vi "Main.vi"() -> ()   [LabVIEW 2014]
uses:
  <vilib>/userdefined/High Color/IMAQdx.ctl
  <vilib>/myRIO/Common/Instrument Driver Framework/myRIO v1.0/UART/vis/myRIO v1.0 Close UART.vi
  <vilib>/addons/control/pid/pid.llb/PID (DBL).vi
  <vilib>/myRIO/Common/Instrument Driver Framework/Utilities/vis/FPGA Ref Manager.vi
  <vilib>/myRIO/Common/Instrument Driver Framework/myRIO v1.0/myRIO v1.0 Reset FPGA.vi
  <vilib>/myRIO/Common/Instrument Driver Framework/myRIO v1.0/IRQ/vis/myRIO v1.0 IRQ Info FGV.vi
  <vilib>/myRIO/Common/Instrument Driver Framework/myRIO v1.0/IRQ/vis/myRIO v1.0 Timer IRQ Info FGV.vi
  <vilib>/myRIO/Common/Instrument Driver Framework/myRIO v1.0/IRQ/vis/myRIO v1.0 ISR Agent.vi
  <vilib>/vision/driver/NI_Vision_Acquisition_Software.lvlib
  <vilib>/vision/NI_Vision_Development_Module.lvlib
  <vilib>/myRIO/Instrument Drivers/Utilities/Utilities.lvlib
  <vilib>/addons/control/pid/NI_PID_pid.lvlib
panel:
  out "pwm elbow":dbl
  in  "PID gains 2":T1={"proportional gain (Kc)"=1.0, "integral time (Ti, min)"=0.01, "derivative time (Td, min)"=0.0} {"derivative time (Td, min)" format="%.3f"; "integral time (Ti, min)" format="%.3f"; "proportional gain (Kc)" format="%.3f"}
  out "pid elbow":dbl
  out "Boolean 4":bool
  out "Boolean 3":bool
  out "Numeric 2":dbl
  out "Numeric":dbl
  out "pid base":dbl
  out "pwm base":dbl
  out "Boolean 2":bool
  out "Boolean":bool
  in  "PID gains":T1={"proportional gain (Kc)"=0.001, "integral time (Ti, min)"=-0.001, "derivative time (Td, min)"=0.001} {"derivative time (Td, min)" format="%.3f"; "integral time (Ti, min)" format="%.3f"; "proportional gain (Kc)" format="%.3f"}
  out "error out":errorcluster
  in  "Red or Hue Range":cluster{dbl, dbl}(slide)={0.0, 73.71681415929203} scale=0.0..255.0
  in  "Green or Sat Range":cluster{dbl, dbl}(slide)={159.1907514450867, 255.0} scale=0.0..255.0
  out "live feed":T2(plugin-control)
  out "Number of Objects":i32
  out "Found Objects":T3(array[cluster]) {"Aspect Ratio" format="%.2f"; "Orientation" format="%.2f"; "Area" format="%.2f"; "Object Center"."Y" format="%.2f"; "Object Center"."X" format="%.2f"}
  out "Largest Area":sgl
  out "Object Info":T4
  in  "Blue or Luma or Val or Inten Range":cluster{dbl, dbl}(slide)={34.638728323699425, 255.0} scale=0.0..255.0
  in  "stop":bool
  out "threshold":T2(plugin-control)
  in  "Number of Erosion":i32=2
  out "centroid x-displacement":sgl
  out "centroid y-displacement":sgl
  out "Left x-displacement":i32
  out "Top y-displacement":i32
  out "Right x-displacement":i32
  out "Bottom y-displacement":i32
  out "object width":i32
  out "object height":i32
  out "duty cycle of wrist motor":dbl format="%.2f"
  out "box area":dbl
  in  "Session In":T5
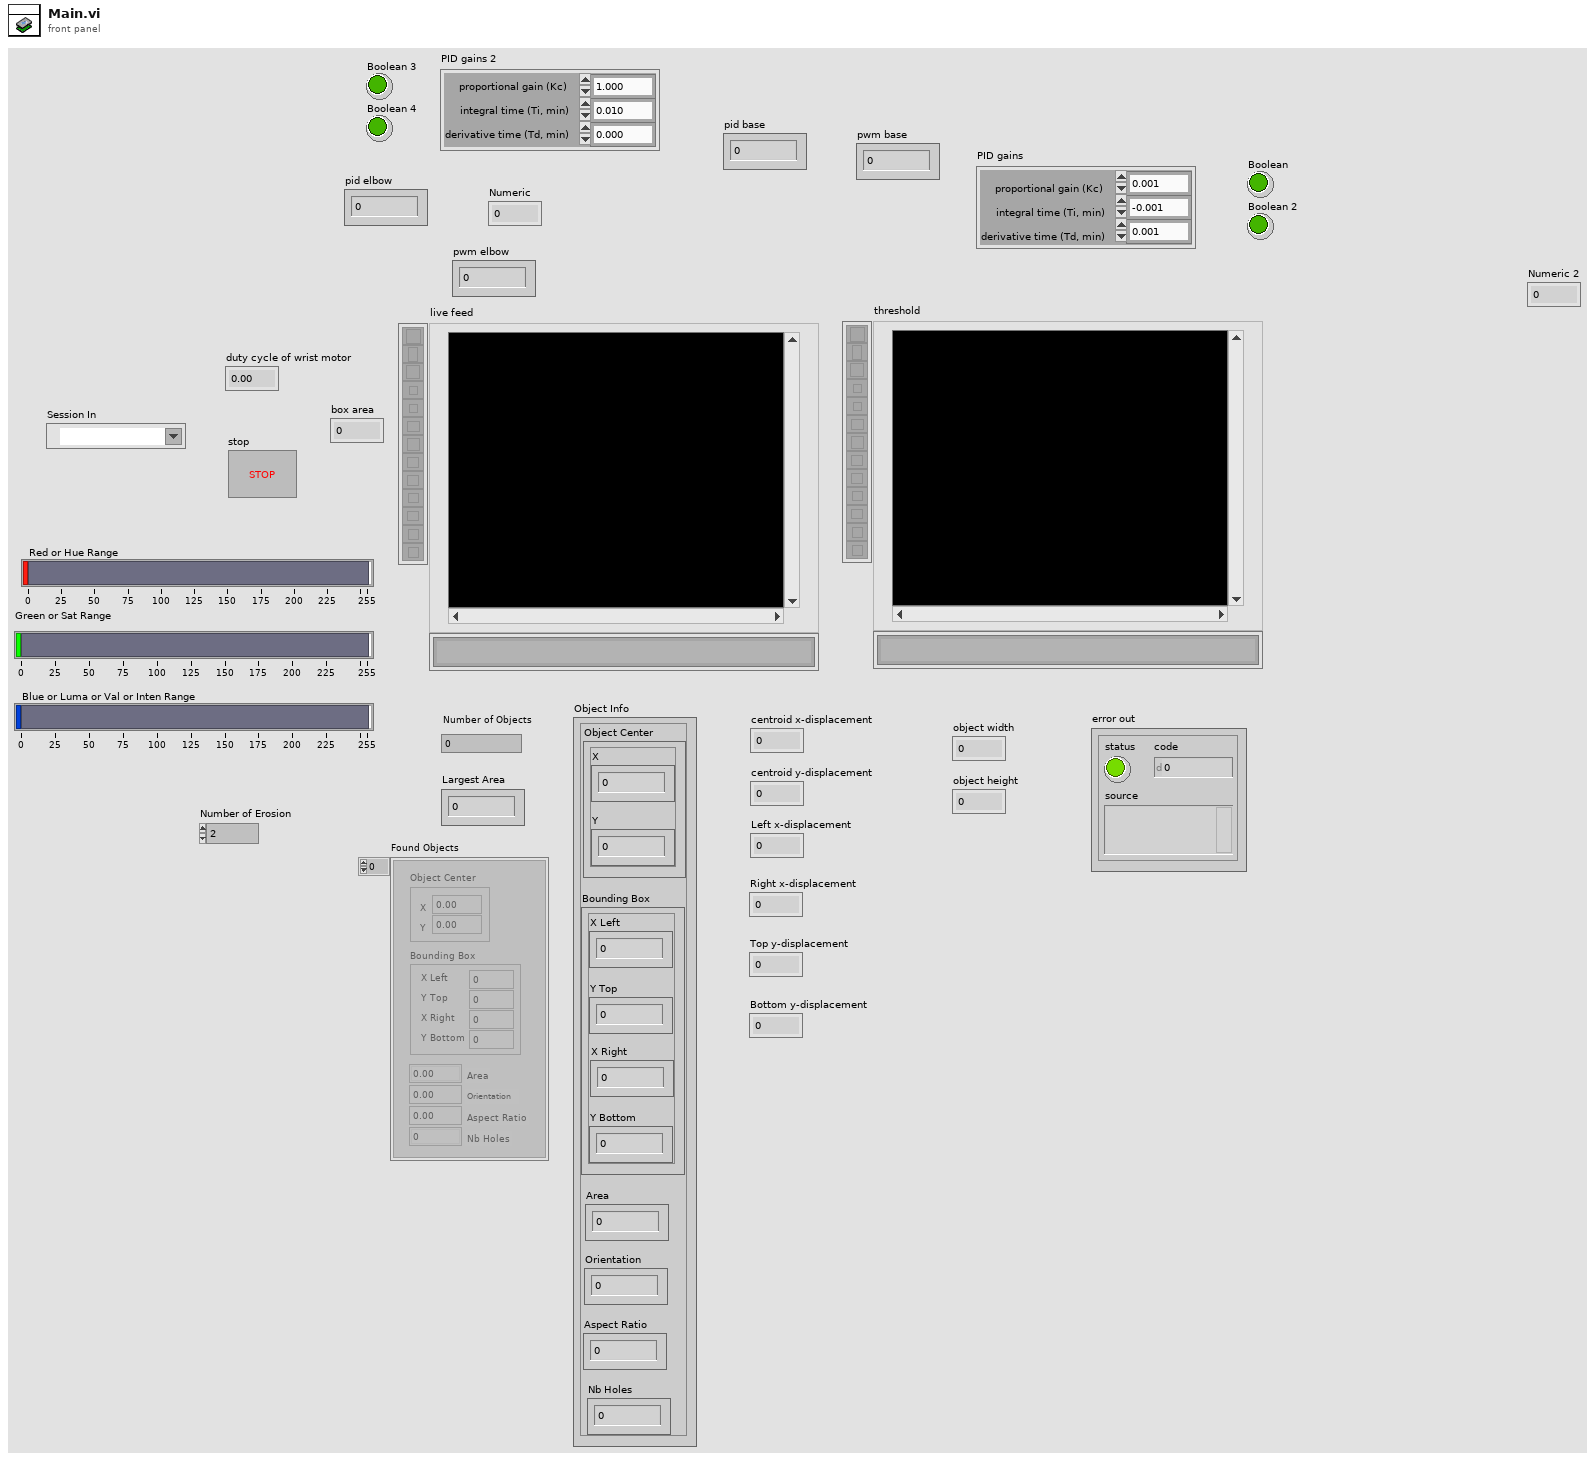
[diagram p1: front panel]
types:
  T1 = cluster{"proportional gain (Kc)":dbl, "integral time (Ti, min)":dbl, "derivative time (Td, min)":dbl}
  T2 = typedef "IMAQ Image.ctl" = refnum<image>
  T3 = cluster{"Object Center":cluster{"X":sgl, "Y":sgl}, "Bounding Box":cluster{"X Left":i32, "Y Top":i32, "X Right":i32, "Y Bottom":i32}, "Area":sgl, "Orientation":sgl, "Aspect Ratio":sgl, "Nb Holes":i32}[]
  T4 = cluster{"Object Center":cluster{"X":sgl, "Y":sgl}, "Bounding Box":cluster{"X Left":i32, "Y Top":i32, "X Right":i32, "Y Bottom":i32}, "Area":sgl, "Orientation":sgl, "Aspect Ratio":sgl, "Nb Holes":i32}
  T5 = typedef "IMAQdx.ctl" = refnum<k21>
  T6 = cluster{"Objects":u16, "Threshold":i32, "Reject Border":bool, "Fill Holes":bool, "Min Object Size":bool, "Min Size":i32, "Max Object Size":bool, "Max Size":i32, "Show Search Area":bool, "Show Center":bool, "Show Bounding Box":bool}
  T7 = typedef "Image Type" = u32
  T8 = cluster{"X Left":i32, "Y Top":i32, "X Right":i32, "Y Bottom":i32}
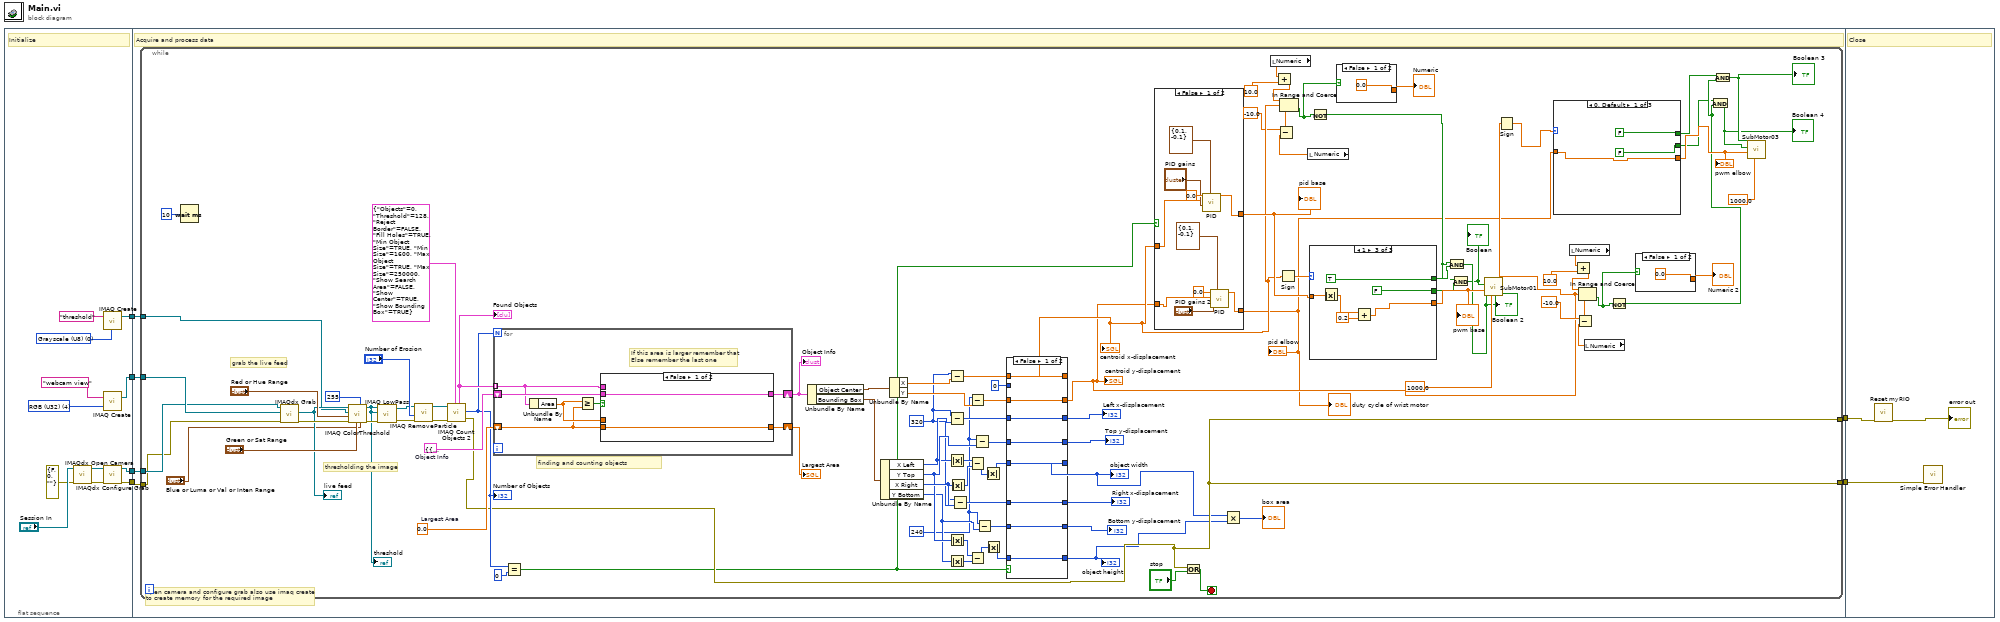
[diagram p0: block diagram]
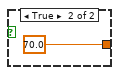
[diagram p2: hidden frame]
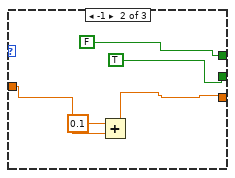
[diagram p3: hidden frame]
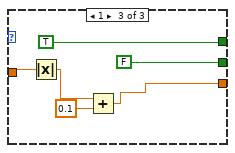
[diagram p4: hidden frame]
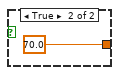
[diagram p5: hidden frame]
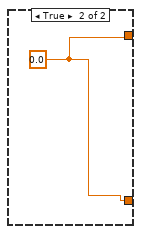
[diagram p6: hidden frame]
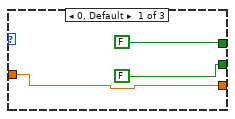
[diagram p7: hidden frame]
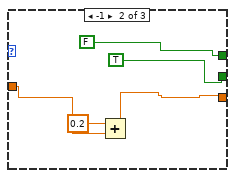
[diagram p8: hidden frame]
diagram:
  n1 = flat-sequence {
    tunnel: [w16] -> w6
    tunnel: [w13] -> w5
    tunnel: [w10] -> w4
    tunnel: [w7] -> w3
    tunnel: [w20] -> w2
    tunnel: w6 -> [w23]
    tunnel: [w19] -> w1
    tunnel: w5 -> [w22]
    tunnel: w4 -> [w21]
    tunnel: w3 -> [w24]
    tunnel: w2 -> [w188]
    tunnel: w1 -> [w186]
    frame #0 {
      w8 = T7 0 items=["Grayscale (U8)", "Grayscale (I16)", "Grayscale (SGL)", "Complex (CSG)", "RGB (U32)", "HSL (U32)", "RGB (U64)", "Grayscale (U16)"] ("Image Type")
      w17 = T7 4 items=["Grayscale (U8)", "Grayscale (I16)", "Grayscale (SGL)", "Complex (CSG)", "RGB (U32)", "HSL (U32)", "RGB (U64)", "Grayscale (U16)"] ("Image Type")
      # "Initialize"
      n2 = call <vilib>:"IMAQdx Open Camera.vi"("error in"=errorcluster {"status"=FALSE, "code"=0, "source"=""} ("error out"), "Session In"="Session In") -> ("error out"=w12:errorcluster, "Session Out"=w14:T5)  [unwired: 8 in]
      n3 = call "IMAQ Create"("Image Name"="threshold", "Image Type"=w8) -> ("New Image"=w7:T2)  [unwired: 3 in, 1 out]
      n4 = call "IMAQ Create"("Image Name"="webcam view", "Image Type"=w17) -> ("New Image"=w16:T2)  [unwired: 3 in, 1 out]
      n5 = call <vilib>:"IMAQdx Configure Grab.vi"("error in"=w12, "Session In"=w14) -> ("error out"=w10:errorcluster, "Session Out"=w13:T5)  [unwired: 8 in]
    }
    frame #1 {
      # "open camera and configure grab also use imaq create \nto create memory for the required image"
      # "Acquire and process data"
      n6 = while {
        tunnel: w24 -> [w71]
        tunnel: w23 -> [w70]
        tunnel: w22 -> [w69]
        tunnel: w21 -> [w68]
        tunnel: [w65] -> w20
        tunnel: [w65] -> w19
        stop <- w66 stop-if-true
        w76 = 240
        w78 = 320
        w116 = T4 {"Object Center"={"X"=0.0, "Y"=0.0}, "Bounding Box"={"X Left"=0, "Y Top"=0, "X Right"=0, "Y Bottom"=0}, "Area"=0.0, "Orientation"=0.0, "Aspect Ratio"=0.0, "Nb Holes"=0}  # Object Info
        w115 = sgl 0.0  # Largest Area
        # "finding and counting objects"
        # "thresholding the image"
        # "grab the live feed"
        n7 = Wait (ms)(milliseconds to wait=u32 10) -> ()  [unwired: 1 out]
        n8 = call <vilib>:"IMAQdx Grab.vi"("error in"=w68, "Image In"=w70, "Session In"=w69) -> ("error out"=w122:errorcluster, "Image Out"=w118:T2)  [unwired: 5 in, 2 out]
        "live feed" <- w118
        n9 = call "IMAQ ColorThreshold"("Blue or Luma or Val or Inten Range"="Blue or Luma or Val or Inten Range", "Replace Value"=255, "Green or Sat Range"="Green or Sat Range", "error in (no error)"=w122, "Red or Hue Range"="Red or Hue Range", "Image Dst"=w71, "Image Src"=w118) -> ("error out"=w112:errorcluster, "Image Dst Out"=w111:T2)  [unwired: 3 in]
        "threshold" <- w111
        n10 = call "IMAQ LowPass"("Image Src"=w111, "Image Mask"=w111, "error in (no error)"=w112) -> ("Image Dst Out"=w73:T2, "error out"=w75:errorcluster)  [unwired: 4 in]
        n11 = call "IMAQ RemoveParticle"("error in (no error)"=w75, "Number of Erosion"="Number of Erosion", "Image Src"=w73) -> ("error out"=w74:errorcluster, "Image Dst Out"=w72:T2)  [unwired: 7 in]
        n12 = call "IMAQ Count Objects 2"("Settings"=T6 {"Objects"=0, "Threshold"=128, "Reject Border"=FALSE, "Fill Holes"=TRUE, "Min Object Size"=TRUE, "Min Size"=1600, "Max Object Size"=TRUE, "Max Size"=250000, "Show Search Area"=FALSE, "Show Center"=TRUE, "Show Bounding Box"=TRUE}, "error in (no error)"=w74, "Image"=w72) -> ("error out"=w65:errorcluster, "Number of Objects"=w104:i32, "Objects"=w117:T3)  [unwired: 4 in, 2 out]
        "Number of Objects" <- w104
        "Found Objects" <- w117
        n13 = for {
          N: w104 -> [_]
          tunnel: w117 -> [w178] mode=indexing
          shift-right: [w181] -> w114
          shift-left: w115 -> [w175]
          shift-right: [w180] -> w110
          shift-left: w116 -> [w179]
          # "If this area is larger remember that\nElse remember the last one"
          n14 = Unbundle By Name(w178) -> ("Area"=w177:sgl)
          n15 = Greater Or Equal?(x=w177, y=w175) -> (x >= y?=w176:bool)
          n16 = case shown="False" w176 {
            tunnel: [w183 w185] -> w181
            tunnel: w177 -> [_ w185]
            tunnel: w175 -> [w183 _]
            tunnel: [w182 w184] -> w180
            tunnel: w179 -> [w182 _]
            tunnel: w178 -> [_ w184]
            frame False {
            }
            frame True {
            }
          }
        }
        "Largest Area" <- w114
        "Object Info" <- w110
        n17 = Equal?(x=w104, y=0) -> (x = y?=w58:bool)
        n18 = Unbundle By Name(w110) -> ("Object Center"=w109:cluster{"X":sgl, "Y":sgl}, "Bounding Box"=w107:T8)
        n19 = Unbundle By Name(w107) -> ("X Left"=w79:i32, "Y Top"=w80:i32, "X Right"=w81:i32, "Y Bottom"=w77:i32)
        n20 = Unbundle By Name(w109) -> ("X"=w83:sgl, "Y"=w82:sgl)
        n21 = Subtract(x=w78, y=w83) -> (x-y=w97:sgl)
        n22 = Subtract(x=w78, y=w79) -> (x-y=w95:i32)
        n23 = Absolute Value(x=w79) -> (abs(x)=w89:i32)
        n24 = Absolute Value(x=w80) -> (abs(x)=w91:i32)
        n25 = Absolute Value(x=w77) -> (abs(x)=w90:i32)
        n26 = Absolute Value(x=w81) -> (abs(x)=w88:i32)
        n27 = Subtract(x=w78, y=w81) -> (x-y=w93:i32)
        n28 = Subtract(x=w76, y=w82) -> (x-y=w96:sgl)
        n29 = Subtract(x=w89, y=w88) -> (x-y=w87:i32)
        n30 = Subtract(x=w91, y=w90) -> (x-y=w85:i32)
        n31 = Subtract(x=w76, y=w80) -> (x-y=w94:i32)
        n32 = Subtract(x=w76, y=w77) -> (x-y=w92:i32)
        n33 = Absolute Value(x=w87) -> (abs(x)=w86:i32)
        n34 = Absolute Value(x=w85) -> (abs(x)=w84:i32)
        n35 = case shown="False" w58 {
          tunnel: [w173 w174] -> w56
          tunnel: 0 -> [_ w174]
          tunnel: [w172 w174] -> w33
          tunnel: [w171 w174] -> w101
          tunnel: [w169 w174] -> w100
          tunnel: [w170 w174] -> w99
          tunnel: [w168 w174] -> w98
          tunnel: w97 -> [w173 _]
          tunnel: w96 -> [w172 _]
          tunnel: w95 -> [w171 _]
          tunnel: w94 -> [w170 _]
          tunnel: w93 -> [w169 _]
          tunnel: w92 -> [w168 _]
          tunnel: [w167 w174] -> w63
          tunnel: w86 -> [w167 _]
          tunnel: [w166 w174] -> w62
          tunnel: w84 -> [w166 _]
          frame False {
          }
          frame True {
          }
        }
        "centroid x-displacement" <- w56
        "centroid y-displacement" <- w33
        "Left x-displacement" <- w101
        "Top y-displacement" <- w99
        "Right x-displacement" <- w100
        "Bottom y-displacement" <- w98
        "object width" <- w63
        "object height" <- w62
        n36 = case shown="False" w58 {
          tunnel: [w142 w151] -> w32
          tunnel: w33 -> [w145 _]
          tunnel: [w143 w151] -> w57
          tunnel: w56 -> [w144 _]
          frame False {
            n37 = call-poly <vilib>:"PID.vi"("output range"=cluster{"output high":dbl, "output low":dbl} {"output high"=0.1, "output low"=-0.1}, "PID gains"="PID gains", "process variable"=w144, "setpoint"=0.0) -> ("output"=w143:dbl)  [unwired: 6 in, 1 out]
            n38 = call-poly <vilib>:"PID.vi"("output range"=cluster{"output high":dbl, "output low":dbl} {"output high"=0.1, "output low"=-0.1}, "PID gains"="PID gains 2", "process variable"=w145, "setpoint"=0.0) -> ("output"=w142:dbl)  [unwired: 6 in, 1 out]
          }
          frame True {
            w151 = 0.0
          }
        }
        "duty cycle of wrist motor" <- w32
        "pid base" <- w57
        "pid elbow" <- w32
        n39 = Or(x=w65, y="stop") -> (x .or. y?=w66:bool)
        n40 = Multiply(x=w63, y=w62) -> (x*y=→"box area":i32)
        n41 = local read "Numeric"() -> (w48:dbl)
        n42 = Add(x=w48, y=10.0 ("upper limit")) -> (x+y=w47:dbl)
        n43 = Sign(1:w56) -> (0:w61:sgl)
        n44 = local read "Numeric"() -> (w45:dbl)
        n45 = Subtract(x=-10.0 ("lower limit"), y=w45) -> (x-y=w44:dbl)
        n46 = In Range and Coerce(upper limit=w47, x=w56, lower limit=w44) -> (In Range?=w50:bool)  [unwired: 1 out]
        n47 = case shown="1" w61 {
          tunnel: [FALSE FALSE TRUE] -> w54
          tunnel: [FALSE TRUE FALSE] -> w53
          tunnel: [w152 w156 w162] -> w59
          tunnel: w57 -> [w152 w155 w160]
          frame 0, Default {
          }
          frame -1 {
            n48 = Add(x=0.2, y=w155) -> (x+y=w156:dbl)
          }
          frame 1 {
            n49 = Absolute Value(x=w160) -> (abs(x)=w161:dbl)
            n50 = Add(x=w161, y=0.2) -> (x+y=w162:dbl)
          }
        }
        "pwm base" <- w59
        n51 = Not(x=w50) -> (.not. x?=w51:bool)
        n52 = case shown="False" w50 {
          tunnel: [0.0 70.0] -> w43
          frame False {
          }
          frame True {
          }
        }
        "Numeric" <- w43
        n53 = And(x=w51, y=w54) -> (x .and. y?=w55:bool)
        "Boolean 2" <- w55
        n54 = And(x=w51, y=w53) -> (x .and. y?=w52:bool)
        "Boolean" <- w52
        n55 = call "SubMotor01.vi"("Frequency [Hz]"=1000.0, "Duty Cycle"=w59, "A/DIO14 (Pin 32)"=w52, "A/DIO15 (Pin 34)"=w55) -> ()  [unwired: 5 in, 3 out]
        n56 = Sign(1:w33) -> (0:w42:sgl)
        n57 = case shown="0, Default" w42 {
          tunnel: [FALSE FALSE TRUE] -> w28
          tunnel: [FALSE TRUE FALSE] -> w27
          tunnel: [w125 w129 w135] -> w30
          tunnel: w32 -> [w125 w128 w133]
          frame 0, Default {
          }
          frame -1 {
            n58 = Add(x=0.1, y=w128) -> (x+y=w129:dbl)
          }
          frame 1 {
            n59 = Absolute Value(x=w133) -> (abs(x)=w134:dbl)
            n60 = Add(x=w134, y=0.1) -> (x+y=w135:dbl)
          }
        }
        "pwm elbow" <- w30
        n61 = local read "Numeric"() -> (w39:dbl)
        n62 = Add(x=w39, y=10.0 ("upper limit")) -> (x+y=w38:dbl)
        n63 = local read "Numeric"() -> (w36:dbl)
        n64 = Subtract(x=-10.0 ("lower limit"), y=w36) -> (x-y=w35:dbl)
        n65 = In Range and Coerce(upper limit=w38, x=w33, lower limit=w35) -> (In Range?=w41:bool)  [unwired: 1 out]
        n66 = Not(x=w41) -> (.not. x?=w29:bool)
        n67 = case shown="False" w41 {
          tunnel: [0.0 70.0] -> w34
          frame False {
          }
          frame True {
          }
        }
        "Numeric 2" <- w34
        n68 = And(x=w27, y=w29) -> (x .and. y?=w25:bool)
        "Boolean 4" <- w25
        n69 = And(x=w28, y=w29) -> (x .and. y?=w26:bool)
        "Boolean 3" <- w26
        n70 = call "SubMotor03.vi"("Frequency [Hz]"=1000.0, "Duty Cycle"=w30, "A/DIO1 (Pin 13)"=w25, "A/DIO2 (Pin 15)"=w26) -> ()  [unwired: 5 in, 3 out]
      }
    }
    frame #2 {
      # "Close"
      n71 = call <vilib>:"Reset myRIO.vi"("error in (no error)"=w188) -> ("error out"=→"error out":errorcluster)  [unwired: 10 in]
      n72 = call <vilib>:"Simple Error Handler.vi"("error in (no error)"=w186) -> ()  [unwired: 4 in, 5 out]
    }
  }
